vi "Fast Query Reply.vi"(6 "Field Names":string[](array[string]), 8 "error in (no error)":errorcluster, 9 "Meta Data":variant, 10 "Return Data":string[][](array[string]), 11 "Module ID":i32=-1) -> (0 "error out":errorcluster)   [LabVIEW 2014, in "DB_CONNECTOR.lvlib"]
doc: "The database reply from a (asynchonous) \"Fast Query\".\n_____\nCreated using Delacor QMH Event Scripter 4.1.0.80."
uses:
  DB_CONNECTOR.lvlib
  Fast Query Reply Argument--cluster.ctl
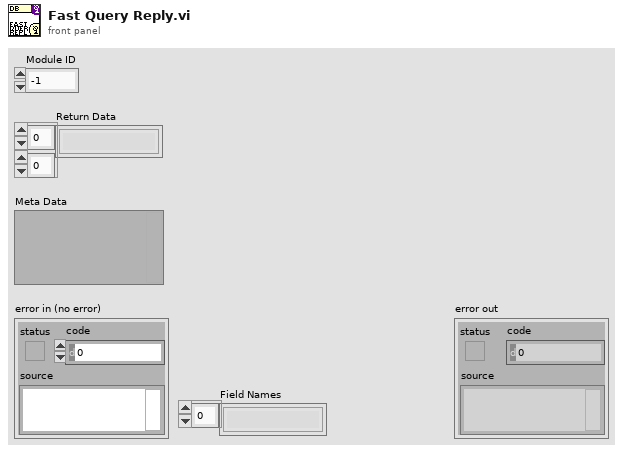
[diagram p1: front panel]
types:
  T1 = typedef "DB_CONNECTOR.lvlib/Fast Query Reply Argument--cluster.ctl" = cluster{"Module ID":i32, "Return Data":string[][], "Meta Data":variant, "Field Names":string[]}
  T2 = typedef "DB_CONNECTOR.lvlib/Broadcast Events--cluster.ctl" = cluster{"Module Did Init":refnum<user-event>, "Status Updated":refnum<user-event>, "Error Reported":refnum<user-event>, "Module Did Stop":refnum<user-event>, "Update Module Execution Status":refnum<user-event>, "Fast Query Reply":refnum<user-event>}
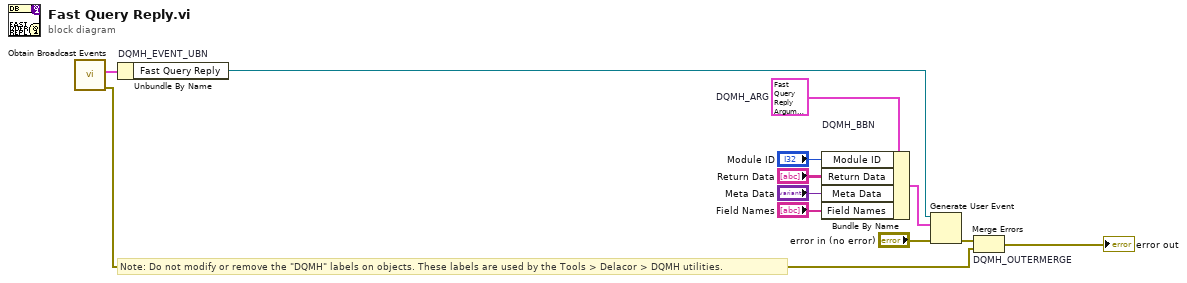
[diagram p0: block diagram]
diagram:
  w7 = T1 {"Module ID"=-1, "Return Data"=[], "Meta Data"=variant, "Field Names"=[]}  # DQMH_ARG
  # "Note: Do not modify or remove the \"DQMH\" labels on objects. These labels are used by the Tools > Delacor > DQMH utilities."
  n1 = call "Obtain Broadcast Events.vi"() -> ("error out"=w2:errorcluster, "DB_CONNECTOR Broadcast Events"=w1:T2)  [unwired: 10 in]
  n2 = Unbundle By Name "DQMH_EVENT_UBN"(w1) -> ("Fast Query Reply"=w9:refnum<user-event>)
  n3 = Bundle By Name "DQMH_BBN"(cluster=w7, "Module ID"="Module ID", "Return Data"="Return Data", "Meta Data"="Meta Data", "Field Names"="Field Names") -> (w10:T1)
  n4 = Generate User Event(user event=w9, event data cluster=w10, error in="error in (no error)") -> (error out=w8:errorcluster)  [unwired: 1 in, 1 out]
  n5 = Merge Errors "DQMH_OUTERMERGE"(w8, w2) -> (→"error out":errorcluster)
